vi "log analysis_gps.vi"() -> ()   [LabVIEW 2018] (continued)
0.1010,5.0842,0f000001,0*696fd9b1\n\t", "DUALANTENNAHEADINGA,USB3,0,48.5,FINESTEERING,2107,283554.100,02000000,d426,15824;INSUFFICIENT_OBS,NONE,-1.000000000,0.000000000,0.000000000,0.0,0.000000000,0.000000000,\"631T\",13,4,4,3,04,00,20,02*de32c05b\n\t", "INSPVAXA,USB3,0,51.0,FINESTEERING,2107,283554.600,02000000,471d,15824;INS_ALIGNMENT_COMPLETE,INS_RTKFIXED,37.37125848358,126.72235217781,7.9795,22.3000,0.0223,-0.2763,0.0124,-2.892819267,-0.280095971,268.699067349,0.4384,0.2951,0.5740,0.1126,0.0925,0.0783,0.0963,0.1010,5.0853,0f000001,0*82db867f\n\t", "DUALANTENNAHEADINGA,USB3,0,47.0,FINESTEERING,2107,283555.100,02000000,d426,15824;INSUFFICIENT_OBS,NONE,-1.000000000,0.000000000,0.000000000,0.0,0.000000000,0.000000000,\"631T\",14,4,4,3,04,00,20,03*a9c2070c\n\t", "INSPVAXA,USB3,0,47.0,FINESTEERING,2107,283555.600,02000000,471d,15824;INS_ALIGNMENT_COMPLETE,INS_RTKFIXED,37.37125853353,126.72234893237,7.9755,22.3000,0.0216,-0.2860,0.0144,-2.819506648,-0.407770491,269.082070244,0.4381,0.2951,0.5741,0.1126,0.0924,0.0783,0.0963,0.1010,5.0867,0f000001,0*4971d182\n\t", "INSPVAXA,USB3,0,45.0,FINESTEERING,2107,283556.100,02000000,471d,15824;INS_ALIGNMENT_COMPLETE,INS_RTKFIXED,37.37125856914,126.72234737250,7.9744,22.3000,0.0229,-0.2921,0.0135,-2.758204349,-0.398675406,269.289539292,0.4378,0.2952,0.5740,0.1126,0.0924,0.0783,0.0962,0.1010,5.0883,0f000001,0*04f4864c\n\t", "DUALANTENNAHEADINGA,USB3,0,45.0,FINESTEERING,2107,283556.600,02000000,d426,15824;INSUFFICIENT_OBS,NONE,-1.000000000,0.000000000,0.000000000,0.0,0.000000000,0.000000000,\"631T\",14,4,4,3,04,00,20,03*1b8bbdb9\n\t", "DUALANTENNAHEADINGA,USB3,0,45.0,FINESTEERING,2107,283557.100,02000000,d426,15824;INSUFFICIENT_OBS,NONE,-1.000000000,0.000000000,0.000000000,0.0,0.000000000,0.000000000,\"631T\",15,4,4,3,04,00,20,03*6d1923ae\n\t", "DUALANTENNAHEADINGA,USB3,0,46.5,FINESTEERING,2107,283557.600,02000000,d426,15824;INSUFFICIENT_OBS,NONE,-1.000000000,0.000000000,0.000000000,0.0,0.000000000,0.000000000,\"631T\",14,4,4,3,04,00,20,03*8fe42440\n\t", "DUALANTENNAHEADINGA,USB3,0,46.5,FINESTEERING,2107,283558.100,02000000,d426,15824;INSUFFICIENT_OBS,NONE,-1.000000000,0.000000000,0.000000000,0.0,0.000000000,0.000000000,\"631T\",11,4,4,3,04,00,20,02*089ab1fe\n\t", "INSPVAXA,USB3,0,47.5,FINESTEERING,2107,283558.600,02000000,471d,15824;INS_ALIGNMENT_COMPLETE,INS_RTKFIXED,37.37125886562,126.72233975708,7.9685,22.3000,0.0526,-0.2759,0.0211,-2.409557071,-0.340107874,269.967780628,0.4378,0.2950,0.5739,0.1125,0.0924,0.0783,0.0962,0.1009,5.0913,0f000001,0*5e667246\n\t", "DUALANTENNAHEADINGA,USB3,0,47.5,FINESTEERING,2107,283559.100,02008000,d426,15824;INSUFFICIENT_OBS,NONE,-1.000000000,0.000000000,0.000000000,0.0,0.000000000,0.000000000,\"631T\",9,4,4,3,04,00,20,03*5bfaaf18\n\t", "DUALANTENNAHEADINGA,USB3,0,51.0,FINESTEERING,2107,283559.600,02008000,d426,15824;INSUFFICIENT_OBS,NONE,-1.000000000,0.000000000,0.000000000,0.0,0.000000000,0.000000000,\"631T\",11,4,4,3,04,00,20,03*aa74f950\n\t", "DUALANTENNAHEADINGA,USB3,0,43.5,FINESTEERING,2107,283560.100,02008000,d426,15824;INSUFFICIENT_OBS,NONE,-1.000000000,0.000000000,0.000000000,0.0,0.000000000,0.000000000,\"631T\",12,4,4,3,04,00,20,02*918dc314\n\t", "INSPVAXA,USB3,0,43.5,FINESTEERING,2107,283560.600,02008000,471d,15824;INS_ALIGNMENT_COMPLETE,INS_RTKFIXED,37.37125922477,126.72233331539,7.9711,22.3000,0.0461,-0.3029,0.0142,-2.105523961,0.098116504,270.318274292,0.4374,0.2952,0.5740,0.1125,0.0925,0.0783,0.0962,0.1009,5.0942,0f000001,0*4e7a44d6\n\t", "DUALANTENNAHEADINGA,USB3,0,45.0,FINESTEERING,2107,283561.600,02008000,d426,15824;INSUFFICIENT_OBS,NONE,-1.000000000,0.000000000,0.000000000,0.0,0.000000000,0.000000000,\"631T\",11,4,4,3,04,00,20,03*333d7c31\n\t", "DUALANTENNAHEADINGA,USB3,0,45.0,FINESTEERING,2107,283562.100,02008000,d426,15824;INSUFFICIENT_OBS,NONE,-1.000000000,0.000000000,0.000000000,0.0,0.000000000,0.000000000,\"631T\",10,4,4,3,04,00,20,03*9e1feb94\n\t", "DUALANTENNAHEADINGA,USB3,0,49.5,FINESTEERING,2107,283562.600,02008000,d426,15824;INSUFFICIENT_OBS,NONE,-1.000000000,0.000000000,0.000000000,0.0,0.000000000,0.000000000,\"631T\",11,4,4,3,04,00,20,03*0e8972e5\n\t", "DUALANTENNAHEADINGA,USB3,0,49.5,FINESTEERING,2107,283563.100,02008000,d426,15824;INSUFFICIENT_OBS,NONE,-1.000000000,0.000000000,0.000000000,0.0,0.000000000,0.000000000,\"631T\",12,4,4,3,04,00,20,03*0cafea03\n\t", "DUALANTENNAHEADINGA,USB3,0,49.5,FINESTEERING,2107,283563.600,02000000,d426,15824;INSUFFICIENT_OBS,NONE,-1.000000000,0.000000000,0.000000000,0.0,0.000000000,0.000000000,\"631T\",11,4,4,3,04,00,20,03*75c2f29d\n\t", "DUALANTENNAHEADINGA,USB3,0,46.5,FINESTEERING,2107,283564.100,02000000,d426,15824;INSUFFICIENT_OBS,NONE,-1.000000000,0.000000000,0.000000000,0.0,0.000000000,0.000000000,\"631T\",12,4,4,3,04,00,20,03*b22ee873\n\t", "DUALANTENNAHEADINGA,USB3,0,46.5,FINESTEERING,2107,283564.600,02000000,d426,15824;INSUFFICIENT_OBS,NONE,-1.000000000,0.000000000,0.000000000,0.0,0.000000000,0.000000000,\"631T\",13,4,4,3,04,00,20,03*a96472bd\n\t", "DUALANTENNAHEADINGA,USB3,0,46.5,FINESTEERING,2107,283565.100,02000000,d426,15824;INSUFFICIENT_OBS,NONE,-1.000000000,0.000000000,0.000000000,0.0,0.000000000,0.000000000,\"631T\",13,4,4,3,04,00,20,03*08146cf2\n\t", "DUALANTENNAHEADINGA,USB3,0,48.0,FINESTEERING,2107,283565.600,02000000,d426,15824;INSUFFICIENT_OBS,NONE,-1.000000000,0.000000000,0.000000000,0.0,0.000000000,0.000000000,\"631T\",12,4,4,3,04,00,20,03*500b58cb\n\t", "DUALANTENNAHEADINGA,USB3,0,48.0,FINESTEERING,2107,283566.100,02000000,d426,15824;INSUFFICIENT_OBS,NONE,-1.000000000,0.000000000,0.000000000,0.0,0.000000000,0.000000000,\"631T\",13,4,4,3,04,00,20,02*8a2efff8\n\t", "INSPVAXA,USB3,0,47.0,FINESTEERING,2107,283567.150,02000000,471d,15824;INS_ALIGNMENT_COMPLETE,INS_RTKFIXED,37.37126023924,126.72231232835,7.9766,22.3000,0.0196,-0.2915,0.0203,-1.615683840,-0.184237550,266.738571120,0.4436,0.2960,0.5749,0.1133,0.0925,0.0784,0.0962,0.1011,5.1038,0f000001,0*2b446319\n\t", "DUALANTENNAHEADINGA,USB3,0,47.0,FINESTEERING,2107,283567.600,02000000,d426,15824;INSUFFICIENT_OBS,NONE,-1.000000000,0.000000000,0.000000000,0.0,0.000000000,0.000000000,\"631T\",12,4,4,3,04,00,20,02*8ed7ff70\n\t", "DUALANTENNAHEADINGA,USB3,0,47.0,FINESTEERING,2107,283568.100,02000000,d426,15824;INSUFFICIENT_OBS,NONE,-1.000000000,0.000000000,0.000000000,0.0,0.000000000,0.000000000,\"631T\",14,4,4,3,04,00,20,03*aaffec67\n\t", "INSPVAXA,USB3,0,50.5,FINESTEERING,2107,283568.650,02000000,471d,15824;INS_ALIGNMENT_COMPLETE,INS_RTKFIXED,37.37126026613,126.72230748127,7.9785,22.3000,0.0314,-0.2890,0.0136,-1.676303872,0.031387209,266.013991723,0.4441,0.2961,0.5750,0.1133,0.0925,0.0784,0.0962,0.1011,5.1051,0f000001,0*382c449f\n\t", "DUALANTENNAHEADINGA,USB3,0,40.0,FINESTEERING,2107,283569.100,02000000,d426,15824;INSUFFICIENT_OBS,NONE,-1.000000000,0.000000000,0.000000000,0.0,0.000000000,0.000000000,\"631T\",13,4,4,3,04,00,20,02*1cb1745e\n\t", "DUALANTENNAHEADINGA,USB3,0,40.0,FINESTEERING,2107,283569.600,02000000,d426,15824;INSUFFICIENT_OBS,NONE,-1.000000000,0.000000000,0.000000000,0.0,0.000000000,0.000000000,\"631T\",13,4,4,3,04,00,20,03*a71e5e5e\n\t", "INSPVAXA,USB3,0,51.0,FINESTEERING,2107,283570.150,02000000,471d,15824;INS_ALIGNMENT_COMPLETE,INS_RTKFIXED,37.37126027188,126.72230260848,7.9782,22.3000,0.0223,-0.2985,0.0040,-1.310118648,0.027956781,265.914374243,0.4449,0.2965,0.5753,0.1133,0.0927,0.0784,0.0962,0.1011,5.1080,0f000001,0*e4cc9c92\n\t", "INSPVAXA,USB3,0,51.0,FINESTEERING,2107,283570.650,02000000,471d,15824;INS_ALIGNMENT_COMPLETE,INS_RTKFIXED,37.37126026750,126.72230111428,7.9776,22.3000,0.0310,-0.1470,0.0080,-1.255276150,-0.174138807,265.875286689,0.4449,0.2965,0.5753,0.1133,0.0927,0.0784,0.0962,0.1011,5.1080,0f000001,0*fb01e8e4\n\t", "INSPVAXA,USB3,0,50.0,FINESTEERING,2107,283571.150,02000000,471d,15824;INS_ALIGNMENT_COMPLETE,INS_RTKFIXED,37.37126027111,126.72229951558,7.9776,22.3000,-0.0095,-0.3504,-0.0012,-1.130419534,-0.185484043,265.929537810,0.4449,0.2965,0.5753,0.1133,0.0927,0.0784,0.0962,0.1011,5.1080,0f000001,0*20782363\n\t", "DUALANTENNAHEADINGA,USB3,0,50.0,FINESTEERING,2107,283572.100,02000000,d426,15824;INSUFFICIENT_OBS,NONE,0.000000000,0.000000000,0.000000000,0.0,0.000000000,0.000000000,\"\",0,0,0,0,00,00,00,00*5d8535fc\n\t", "DUALANTENNAHEADINGA,USB3,0,52.5,FINESTEERING,2107,283572.600,02000000,d426,15824;INSUFFICIENT_OBS,NONE,0.000000000,0.000000000,0.000000000,0.0,0.000000000,0.000000000,\"\",0,0,0,0,00,00,00,00*859f07a2\n\t", "DUALANTENNAHEADINGA,USB3,0,50.0,FINESTEERING,2107,283573.100,02000000,d426,15824;INSUFFICIENT_OBS,NONE,0.000000000,0.000000000,0.000000000,0.0,0.000000000,0.000000000,\"\",0,0,0,0,00,00,00,00*a797c2ea\n\t", "INSPVAXA,USB3,0,52.0,FINESTEERING,2107,283574.650,02000000,471d,15824;INS_ALIGNMENT_COMPLETE,INS_RTKFIXED,37.37126025479,126.72228822591,7.9861,22.3000,0.0090,-0.3026,-0.0003,-0.524199220,-0.126443269,266.389234836,0.4991,0.3317,0.6500,0.1205,0.0986,0.0804,0.0985,0.1030,5.1132,0f000001,0*c3c99d89\n\t", "INSPVAXA,USB3,0,50.0,FINESTEERING,2107,283575.150,02000000,471d,15824;INS_ALIGNMENT_COMPLETE,INS_RTKFIXED,37.37126023129,126.72228662486,7.9852,22.3000,0.0085,-0.2932,0.0017,-0.596688743,-0.097225443,266.485321234,0.4751,0.3142,0.6322,0.1185,0.0977,0.0789,0.0982,0.1027,5.1147,0f000001,0*e174b094\n\t", "INSPVAXA,USB3,0,50.0,FINESTEERING,2107,283575.650,02000000,471d,15824;INS_ALIGNMENT_COMPLETE,INS_RTKFIXED,37.37126022571,126.72228518067,7.9842,22.3000,-0.0010,-0.2887,0.0210,-0.683424263,-0.147084143,266.527685008,0.4751,0.3142,0.6322,0.1185,0.0977,0.0789,0.0982,0.1027,5.1147,0f000001,0*c2e268d1\n\t", "INSPVAXA,USB3,0,50.0,FINESTEERING,2107,283576.150,02000000,471d,15824;INS_ALIGNMENT_COMPLETE,INS_RTKFIXED,37.37126021633,126.72228346240,7.9840,22.3000,0.0021,-0.2751,0.0114,-0.667866815,-0.315367181,266.708831075,0.4606,0.3053,0.6179,0.1181,0.0979,0.0781,0.0979,0.1024,5.1163,0f000001,0*0ba78e3d\n\t", "INSPVAXA,USB3,0,50.0,FINESTEERING,2107,283576.650,02000000,471d,15824;INS_ALIGNMENT_COMPLETE,INS_RTKFIXED,37.37126022512,126.72228190722,7.9848,22.3000,-0.0006,-0.2994,0.0229,-0.670999350,-0.155338039,266.786409078,0.4606,0.3053,0.6179,0.1181,0.0979,0.0781,0.0979,0.1024,5.1163,0f000001,0*9811c325\n\t", "INSPVAXA,USB3,0,48.5,FINESTEERING,2107,283577.650,02000000,471d,15824;INS_ALIGNMENT_COMPLETE,INS_RTKFIXED,37.37126026454,126.72227868899,7.9856,22.3000,0.0080,-0.2785,0.0173,-0.609374053,-0.154098562,267.060666338,0.4521,0.3012,0.6064,0.1181,0.0980,0.0776,0.0975,0.1023,5.1178,0f000001,0*aa9c2bc5\n\t", "INSPVAXA,USB3,0,51.5,FINESTEERING,2107,283579.150,02000000,471d,15824;INS_ALIGNMENT_COMPLETE,INS_RTKFIXED,37.37126037410,126.72227378516,7.9904,22.3000,0.0163,-0.2830,0.0173,-0.746603441,-0.380752059,267.626447850,0.4463,0.2992,0.5904,0.1180,0.0971,0.0775,0.0966,0.1018,5.1209,0f000001,0*da9a51df\n\t", "INSPVAXA,USB3,0,51.5,FINESTEERING,2107,283579.650,02000000,471d,15824;INS_ALIGNMENT_COMPLETE,INS_RTKFIXED,37.37126042399,126.72227213267,7.9925,22.3000,0.0129,-0.2940,0.0192,-0.723337751,-0.333271037,267.787526970,0.4463,0.2992,0.5904,0.1180,0.0971,0.0775,0.0966,0.1018,5.1209,0f000001,0*2d4308ff\n\t", "INSPVAXA,USB3,0,52.5,FINESTEERING,2107,283580.150,02000000,471d,15824;INS_ALIGNMENT_COMPLETE,INS_RTKFIXED,37.37126049043,126.72227055501,7.9950,22.3000,0.0243,-0.3033,0.0180,-0.573377117,-0.330323438,267.951447700,0.4448,0.2989,0.5852,0.1175,0.0961,0.0776,0.0961,0.1014,5.1224,0f000001,0*65285ec1\n\t", "DUALANTENNAHEADINGA,USB3,0,48.0,FINESTEERING,2107,283581.100,02000000,d426,15824;INSUFFICIENT_OBS,NONE,0.000000000,0.000000000,0.000000000,0.0,0.000000000,0.000000000,\"\",0,0,0,0,00,00,00,00*0d472a41\n\t", "INSPVAXA,USB3,0,48.0,FINESTEERING,2107,283581.650,02000000,471d,15824;INS_ALIGNMENT_COMPLETE,INS_RTKFIXED,37.37126070396,126.72226577509,8.0028,22.3000,0.0230,-0.2933,0.0344,-0.578760971,-0.170041590,268.380757067,0.4441,0.2986,0.5812,0.1168,0.0951,0.0777,0.0958,0.1011,5.1238,0f000001,0*94c5c4b2\n\t", "INSPVAXA,USB3,0,50.0,FINESTEERING,2107,283582.650,02000000,471d,15824;INS_ALIGNMENT_COMPLETE,INS_RTKFIXED,37.37126086300,126.72226255094,8.0114,22.3000,0.0186,-0.2902,0.0297,-0.554451124,-0.113657827,268.567093928,0.4437,0.2982,0.5783,0.1160,0.0941,0.0779,0.0956,0.1009,5.1252,0f000001,0*de1d38ac\n\t", "INSPVAXA,USB3,0,52.0,FINESTEERING,2107,283583.150,02000000,471d,15824;INS_ALIGNMENT_COMPLETE,INS_RTKFIXED,37.37126094107,126.72226089314,8.0147,22.3000,0.0176,-0.2816,0.0224,-0.681553326,-0.108375043,268.657687253,0.4431,0.2976,0.5763,0.1151,0.0933,0.0781,0.0955,0.1007,5.1266,0f000001,0*8a630b8d\n\t", "INSPVAXA,USB3,0,52.0,FINESTEERING,2107,283583.650,02000000,471d,15824;INS_ALIGNMENT_COMPLETE,INS_RTKFIXED,37.37126102705,126.72225926038,8.0174,22.3000,0.0194,-0.3033,0.0147,-0.616207417,-0.286762817,268.672715403,0.4431,0.2976,0.5763,0.1151,0.0933,0.0781,0.0955,0.1007,5.1266,0f000001,0*61848793\n\t", "INSPVAXA,USB3,0,52.0,FINESTEERING,2107,283584.150,02000000,471d,15824;INS_ALIGNMENT_COMPLETE,INS_RTKFIXED,37.37126112105,126.72225762489,8.0208,22.3000,0.0251,-0.2868,0.0143,-0.484996115,-0.348090113,268.682050647,0.4426,0.2969,0.5750,0.1144,0.0927,0.0782,0.0955,0.1006,5.1279,0f000001,0*d30f3e54\n\t", "INSPVAXA,USB3,0,52.0,FINESTEERING,2107,283584.650,02000000,471d,15824;INS_ALIGNMENT_COMPLETE,INS_RTKFIXED,37.37126121621,126.72225620166,8.0227,22.3000,0.0321,-0.0816,0.0199,-0.459149355,-0.498683965,268.628376377,0.4426,0.2969,0.5750,0.1144,0.0927,0.0782,0.0955,0.1006,5.1279,0f000001,0*e5ed7c63\n\t", "INSPVAXA,USB3,0,49.0,FINESTEERING,2107,283585.150,02000000,471d,15824;INS_ALIGNMENT_COMPLETE,INS_RTKFIXED,37.37126129698,126.72225459849,8.0251,22.3000,0.0349,-0.3426,0.0329,-0.569349800,-0.560640511,268.532383253,0.4425,0.2966,0.5744,0.1144,0.0924,0.0784,0.0956,0.1006,5.1294,0f000001,0*4640cbf6\n\t", "INSPVAXA,USB3,0,49.0,FINESTEERING,2107,283585.650,02000000,471d,15824;INS_ALIGNMENT_COMPLETE,INS_RTKFIXED,37.37126137394,126.72225308543,8.0277,22.3000,0.0305,-0.3477,0.0168,-0.707352535,-0.516144165,268.333596331,0.4425,0.2966,0.5744,0.1144,0.0924,0.0784,0.0956,0.1006,5.1294,0f000001,0*ea5ffab2\n\t", "INSPVAXA,USB3,0,50.5,FINESTEERING,2107,283586.150,02000000,471d,15824;INS_ALIGNMENT_COMPLETE,INS_RTKFIXED,37.37126146482,126.72225147889,8.0290,22.3000,0.0318,-0.3117,0.0162,-0.540726540,-0.516678625,268.023762114,0.4406,0.2960,0.5741,0.1134,0.0922,0.0785,0.0957,0.1006,5.1306,0f000001,0*2ae37417\n\t", "INSPVAXA,USB3,0,50.5,FINESTEERING,2107,283586.650,02000000,471d,15824;INS_ALIGNMENT_COMPLETE,INS_RTKFIXED,37.37126154442,126.72224983237,8.0302,22.3000,0.0153,-0.2976,0.0132,-0.405221817,-0.801510438,267.749524136,0.4406,0.2960,0.5741,0.1134,0.0922,0.0785,0.0957,0.1006,5.1306,0f000001,0*889b905c\n\t", "INSPVAXA,USB3,0,48.5,FINESTEERING,2107,283587.150,02000000,471d,15824;INS_ALIGNMENT_COMPLETE,INS_RTKFIXED,37.37126161078,126.72224818389,8.0314,22.3000,0.0135,-0.2861,0.0058,-0.357423684,-1.016170306,267.360005702,0.4401,0.2956,0.5740,0.1128,0.0921,0.0786,0.0958,0.1006,5.1321,0f000001,0*b354eb89\n\t", "DUALANTENNAHEADINGA,USB3,0,48.5,FINESTEERING,2107,283587.600,02000000,d426,15824;INSUFFICIENT_OBS,NONE,0.000000000,0.000000000,0.000000000,0.0,0.000000000,0.000000000,\"\",0,0,0,0,00,00,00,00*3e024a6f\n\t", "INSPVAXA,USB3,0,49.5,FINESTEERING,2107,283588.650,02000000,471d,15824;INS_ALIGNMENT_COMPLETE,INS_RTKFIXED,37.37126174157,126.72224330005,8.0321,22.3000,0.0403,-0.2838,0.0098,-0.134470490,-1.230467800,265.991496419,0.4395,0.2955,0.5741,0.1126,0.0921,0.0786,0.0959,0.1007,5.1336,0f000001,0*86c47da8\n\t", "INSPVAXA,USB3,0,51.5,FINESTEERING,2107,283589.150,02000000,471d,15824;INS_ALIGNMENT_COMPLETE,INS_RTKFIXED,37.37126177483,126.72224169465,8.0328,22.3000,0.0428,-0.2922,0.0200,-0.044724950,-0.991745549,265.567471181,0.4384,0.2954,0.5742,0.1124,0.0922,0.0786,0.0960,0.1008,5.1352,0f000001,0*fd2974d4\n\t", "INSPVAXA,USB3,0,51.5,FINESTEERING,2107,283589.650,02000000,471d,15824;INS_ALIGNMENT_COMPLETE,INS_RTKFIXED,37.37126179570,126.72224014857,8.0325,22.3000,0.0430,-0.3072,0.0249,-0.007617366,-0.680507333,265.196792969,0.4384,0.2954,0.5742,0.1124,0.0922,0.0786,0.0960,0.1008,5.1352,0f000001,0*75474069\n\t", "INSPVAXA,USB3,0,52.0,FINESTEERING,2107,283590.150,02000000,471d,15824;INS_ALIGNMENT_COMPLETE,INS_RTKFIXED,37.37126181306,126.72223852203,8.0321,22.3000,0.0371,-0.3064,0.0221,-0.054866167,-0.319461022,264.939008114,0.4379,0.2954,0.5744,0.1124,0.0922,0.0786,0.0960,0.1008,5.1368,0f000001,0*489db8a8\n\t", "INSPVAXA,USB3,0,52.0,FINESTEERING,2107,283590.650,02000000,471d,15824;INS_ALIGNMENT_COMPLETE,INS_RTKFIXED,37.37126182845,126.72223689511,8.0304,22.3000,0.0329,-0.2983,0.0263,-0.099615260,-0.144209123,264.670119268,0.4379,0.2954,0.5744,0.1124,0.0922,0.0786,0.0960,0.1008,5.1368,0f000001,0*3ff0cb58\n\t", "INSPVAXA,USB3,0,46.5,FINESTEERING,2107,283591.650,02000000,471d,15824;INS_ALIGNMENT_COMPLETE,INS_RTKFIXED,37.37126184009,126.72223359143,8.0280,22.3000,0.0242,-0.3040,0.0144,-0.139661559,-0.269205347,264.433455917,0.4387,0.2955,0.5748,0.1127,0.0923,0.0786,0.0961,0.1009,5.1382,0f000001,0*bb357185\n\t", "INSPVAXA,USB3,0,50.0,FINESTEERING,2107,283592.150,02000000,471d,15824;INS_ALIGNMENT_COMPLETE,INS_RTKFIXED,37.37126183340,126.72223190361,8.0268,22.3000,0.0217,-0.3070,0.0246,-0.250767704,-0.520528814,264.430385141,0.4392,0.2956,0.5751,0.1125,0.0924,0.0786,0.0961,0.1010,5.1393,0f000001,0*012bab97\n\t", "INSPVAXA,USB3,0,50.0,FINESTEERING,2107,283592.650,02000000,471d,15824;INS_ALIGNMENT_COMPLETE,INS_RTKFIXED,37.37126182669,126.72223026122,8.0254,22.3000,0.0249,-0.2956,0.0206,-0.309442980,-0.761179345,264.440443486,0.4392,0.2956,0.5751,0.1125,0.0924,0.0786,0.0961,0.1010,5.1393,0f000001,0*78c848e1\n\t", "INSPVAXA,USB3,0,44.5,FINESTEERING,2107,283593.650,02000000,471d,15824;INS_ALIGNMENT_COMPLETE,INS_RTKFIXED,37.37126179813,126.72222695533,8.0221,22.3000,0.0365,-0.2965,0.0185,-0.369051929,-1.148324870,264.580362201,0.4393,0.2956,0.5754,0.1125,0.0925,0.0786,0.0962,0.1010,5.1403,0f000001,0*8be4a412\n\t", "INSPVAXA,USB3,0,43.0,FINESTEERING,2107,283594.150,02000000,471d,15824;INS_ALIGNMENT_COMPLETE,INS_RTKFIXED,37.37126178881,126.72222531638,8.0209,22.3000,0.0318,-0.2892,0.0117,-0.315197782,-1.127826299,264.669850736,0.4395,0.2956,0.5757,0.1126,0.0925,0.0786,0.0962,0.1010,5.1415,0f000001,0*2d917e72\n\t", "INSPVAXA,USB3,0,43.0,FINESTEERING,2107,283594.650,02000000,471d,15824;INS_ALIGNMENT_COMPLETE,INS_RTKFIXED,37.37126177423,126.72222371508,8.0192,22.3000,0.0303,-0.3062,0.0087,-0.244943668,-0.998392292,264.739545635,0.4395,0.2956,0.5757,0.1126,0.0925,0.0786,0.0962,0.1010,5.1415,0f000001,0*36684632\n\t", "INSPVAXA,USB3,0,48.0,FINESTEERING,2107,283595.150,02000000,471d,15824;INS_ALIGNMENT_COMPLETE,INS_RTKFIXED,37.37126177448,126.72222209651,8.0178,22.3000,0.0339,-0.2977,0.0111,-0.119926645,-0.839441888,264.806746859,0.4396,0.2957,0.5758,0.1127,0.0925,0.0786,0.0962,0.1011,5.1428,0f000001,0*08adb1ac\n\t", "INSPVAXA,USB3,0,48.0,FINESTEERING,2107,283595.650,02000000,471d,15824;INS_ALIGNMENT_COMPLETE,INS_RTKFIXED,37.37126175579,126.72222044305,8.0158,22.3000,0.0315,-0.2901,0.0146,-0.140682450,-0.757275423,264.939327324,0.4396,0.2957,0.5758,0.1127,0.0925,0.0786,0.0962,0.1011,5.1428,0f000001,0*78aa4323\n\t", "INSPVAXA,USB3,0,45.5,FINESTEERING,2107,283596.150,02000000,471d,15824;INS_ALIGNMENT_COMPLETE,INS_RTKFIXED,37.37126174706,126.72221882268,8.0135,22.3000,0.0328,-0.3087,0.0055,-0.159363223,-0.689273148,265.030991748,0.4393,0.2956,0.5759,0.1126,0.0925,0.0785,0.0962,0.1010,5.1440,0f000001,0*bc7a17e4\n\t", "INSPVAXA,USB3,0,47.0,FINESTEERING,2107,283597.650,02000000,471d,15824;INS_ALIGNMENT_COMPLETE,INS_RTKFIXED,37.37126174585,126.72221399388,8.0051,22.3000,0.0336,-0.3137,-0.0021,0.019465738,-0.716944354,265.373596079,0.4393,0.2957,0.5759,0.1127,0.0925,0.0785,0.0962,0.1010,5.1453,0f000001,0*fd9fbe4c\n\t", "INSPVAXA,USB3,0,50.5,FINESTEERING,2107,283598.150,02000000,471d,15824;INS_ALIGNMENT_COMPLETE,INS_RTKFIXED,37.37126175152,126.72221241027,8.0034,22.3000,0.0326,-0.3115,-0.0006,-0.014551220,-0.589641139,265.465982891,0.4393,0.2958,0.5760,0.1127,0.0925,0.0785,0.0962,0.1010,5.1467,0f000001,0*f52d235f\n\t", "INSPVAXA,USB3,0,50.5,FINESTEERING,2107,283598.650,02000000,471d,15824;INS_ALIGNMENT_COMPLETE,INS_RTKFIXED,37.37126174603,126.72221081507,8.0012,22.3000,0.0404,-0.2514,0.0050,0.007312732,-0.531763508,265.590138557,0.4393,0.2958,0.5760,0.1127,0.0925,0.0785,0.0962,0.1010,5.1467,0f000001,0*8824c4d8\n\t", "INSPVAXA,USB3,0,47.5,FINESTEERING,2107,283599.150,02000000,471d,15824;INS_ALIGNMENT_COMPLETE,INS_RTKFIXED,37.37126176062,126.72220950725,7.9992,22.3000,0.0252,-0.3434,0.0010,0.008395245,-0.454774563,265.666808103,0.4392,0.2959,0.5760,0.1129,0.0925,0.0784,0.0962,0.1010,5.1480,0f000001,0*d239d7e1\n\t", "INSPVAXA,USB3,0,49.0,FINESTEERING,2107,283600.150,02000000,471d,15824;INS_ALIGNMENT_COMPLETE,INS_RTKFIXED,37.37126175398,126.72220624813,7.9941,22.3000,0.0263,-0.2975,0.0106,0.196462892,-0.509026578,265.990503300,0.4393,0.2959,0.5760,0.1126,0.0926,0.0784,0.0962,0.1010,5.1489,0f000001,0*3b9f52b7\n\t", "INSPVAXA,USB3,0,49.0,FINESTEERING,2107,283601.150,02000000,471d,15824;INS_ALIGNMENT_COMPLETE,INS_RTKFIXED,37.37126176703,126.72220301301,7.9883,22.3000,0.0322,-0.3028,0.0049,0.082285729,-0.304157914,266.276129441,0.4386,0.2961,0.5760,0.1125,0.0925,0.0784,0.0962,0.1009,5.1498,0f000001,0*cfc5bf1f\n\t", "INSPVAXA,USB3,0,49.0,FINESTEERING,2107,283601.650,02000000,471d,15824;INS_ALIGNMENT_COMPLETE,INS_RTKFIXED,37.37126177893,126.72220143158,7.9847,22.3000,0.0347,-0.3053,0.0090,0.167695581,-0.286452712,266.390208904,0.4386,0.2961,0.5760,0.1125,0.0925,0.0784,0.0962,0.1009,5.1498,0f000001,0*1c01ffd1\n\t", "INSPVAXA,USB3,0,50.0,FINESTEERING,2107,283602.150,02000000,471d,15824;INS_ALIGNMENT_COMPLETE,INS_RTKFIXED,37.37126180222,126.72219979604,7.9806,22.3000,0.0339,-0.2918,-0.0010,0.296365252,-0.279449744,266.507882837,0.4383,0.2960,0.5760,0.1125,0.0926,0.0784,0.0962,0.1009,5.1509,0f000001,0*8cd233aa\n\t", "INSPVAXA,USB3,0,50.5,FINESTEERING,2107,283604.650,02000000,471d,15824;INS_ALIGNMENT_COMPLETE,INS_RTKFIXED,37.37126199805,126.72219243143,7.9649,22.3000,0.0555,0.0695,0.0079,0.560896506,-1.435960650,267.028457385,0.4379,0.2961,0.5759,0.1131,0.0925,0.0784,0.0963,0.1009,5.1528,0f000001,0*81aa449e\n\t", "INSPVAXA,USB3,0,45.0,FINESTEERING,2107,283607.150,02000000,471d,15824;INS_ALIGNMENT_COMPLETE,INS_RTKFIXED,37.37126226214,126.72219256337,7.9563,22.3000,0.0507,-0.0122,0.0067,0.527133772,-1.343948140,267.105174531,0.4402,0.2962,0.5756,0.1140,0.0925,0.0784,0.0963,0.1009,5.1518,0f000001,0*37532215\n\t", "INSPVAXA,USB3,0,45.0,FINESTEERING,2107,283607.650,02000000,471d,15824;INS_ALIGNMENT_COMPLETE,INS_RTKFIXED,37.37126225847,126.72219257288,7.9545,22.3000,0.0487,-0.0117,0.0063,0.526769970,-1.341614130,267.120484585,0.4402,0.2962,0.5756,0.1140,0.0925,0.0784,0.0963,0.1009,5.1518,0f000001,0*097e3cbc\n\t", "INSPVAXA,USB3,0,49.5,FINESTEERING,2107,283619.700,02000000,471d,15824;INS_ALIGNMENT_COMPLETE,INS_RTKFIXED,37.37126206039,126.72216378783,7.9456,22.3000,0.0422,-0.2948,0.0158,1.718323220,-0.193748450,266.266037782,0.4350,0.2957,0.5763,0.1125,0.0925,0.0784,0.0965,0.1009,5.1330,0f000001,0*8635b490\n\t", "INSPVAXA,USB3,0,47.5,FINESTEERING,2107,283622.200,02000000,471d,15824;INS_ALIGNMENT_COMPLETE,INS_RTKFIXED,37.37126217486,126.72215605148,7.9488,22.3000,0.0265,-0.2568,0.0016,0.953197769,-0.264991418,265.735651965,0.4362,0.2956,0.5763,0.1134,0.0927,0.0784,0.0965,0.1010,5.1347,0f000001,0*d1c7aea0\n\t", "INSPVAXA,USB3,0,49.5,FINESTEERING,2107,283623.200,02000000,471d,15824;INS_ALIGNMENT_COMPLETE,INS_RTKFIXED,37.37126215352,126.72215258792,7.9480,22.3000,0.0351,-0.2613,0.0231,0.659350525,-0.553290360,265.516937653,0.4377,0.2954,0.5765,0.1123,0.0931,0.0784,0.0965,0.1010,5.1353,0f000001,0*f37e3ed0\n\t", "INSPVAXA,USB3,0,49.5,FINESTEERING,2107,283625.200,02000000,471d,15824;INS_ALIGNMENT_COMPLETE,INS_RTKFIXED,37.37126210638,126.72214606046,7.9447,22.3000,0.0217,-0.2754,0.0073,0.236515804,-0.792213520,265.180407825,0.4366,0.2950,0.5766,0.1123,0.0931,0.0784,0.0964,0.1010,5.1329,0f000001,0*acc95a4e\n\t", "INSPVAXA,USB3,0,49.5,FINESTEERING,2107,283625.700,02000000,471d,15824;INS_ALIGNMENT_COMPLETE,INS_RTKFIXED,37.37126208247,126.72214443464,7.9445,22.3000,0.0140,-0.2813,0.0048,0.046048670,-0.588797871,265.114785763,0.4366,0.2950,0.5766,0.1123,0.0931,0.0784,0.0964,0.1010,5.1329,0f000001,0*ce0a2a96\n\t", "INSPVAXA,USB3,0,48.0,FINESTEERING,2107,283626.200,02000000,471d,15824;INS_ALIGNMENT_COMPLETE,INS_RTKFIXED,37.37126206372,126.72214280060,7.9445,22.3000,0.0212,-0.2855,0.0048,-0.004156486,-0.311026110,265.065225665,0.4366,0.2949,0.5766,0.1123,0.0931,0.0784,0.0963,0.1010,5.1300,0f000001,0*7442e942\n\t", "INSPVAXA,USB3,0,48.5,FINESTEERING,2107,283627.200,02000000,471d,15824;INS_ALIGNMENT_COMPLETE,INS_RTKFIXED,37.37126201142,126.72213963218,7.9431,22.3000,0.0278,-0.2914,0.0131,-0.197757356,0.430555181,264.900646420,0.4366,0.2949,0.5768,0.1127,0.0931,0.0784,0.0962,0.1009,5.1266,0f000001,0*c875f714\n\t", "INSPVAXA,USB3,0,48.0,FINESTEERING,2107,283628.700,02000000,471d,15824;INS_ALIGNMENT_COMPLETE,INS_RTKFIXED,37.37126191178,126.72213473323,7.9380,22.3000,0.0177,-0.2797,-0.0032,-0.623534384,0.011887408,264.986854356,0.4375,0.2949,0.5768,0.1127,0.0930,0.0784,0.0962,0.1009,5.1221,0f000001,0*2b23c567\n\t", "INSPVAXA,USB3,0,44.0,FINESTEERING,2107,283629.200,02000000,471d,15824;INS_ALIGNMENT_COMPLETE,INS_RTKFIXED,37.37126187751,126.72213308389,7.9364,22.3000,0.0207,-0.2899,-0.0036,-0.719101472,-0.426401600,265.021502859,0.4380,0.2949,0.5768,0.1123,0.0930,0.0784,0.0961,0.1009,5.1171,0f000001,0*92ebbc5f\n\t", "INSPVAXA,USB3,0,44.0,FINESTEERING,2107,283629.700,02000000,471d,15824;INS_ALIGNMENT_COMPLETE,INS_RTKFIXED,37.37126184367,126.72213142920,7.9356,22.3000,0.0231,-0.2981,-0.0100,-0.725013495,-0.732992105,265.121442983,0.4380,0.2949,0.5768,0.1123,0.0930,0.0784,0.0961,0.1009,5.1171,0f000001,0*6a5775b3\n\t", "INSPVAXA,USB3,0,47.0,FINESTEERING,2107,283630.200,02000000,471d,15824;INS_ALIGNMENT_COMPLETE,INS_RTKFIXED,37.37126181957,126.72212981940,7.9352,22.3000,0.0233,-0.2888,-0.0019,-0.675781239,-0.810566304,265.160131093,0.4376,0.2949,0.5768,0.1123,0.0928,0.0784,0.0961,0.1009,5.1128,0f000001,0*27ca04ea\n\t", "INSPVAXA,USB3,0,47.0,FINESTEERING,2107,283630.700,02000000,471d,15824;INS_ALIGNMENT_COMPLETE,INS_RTKFIXED,37.37126178591,126.72212819473,7.9347,22.3000,0.0150,-0.2861,-0.0012,-0.714770911,-0.869266848,265.221494891,0.4376,0.2949,0.5768,0.1123,0.0928,0.0784,0.0961,0.1009,5.1128,0f000001,0*aed2de40\n\t", "INSPVAXA,USB3,0,42.0,FINESTEERING,2107,283631.200,02000000,471d,15824;INS_ALIGNMENT_COMPLETE,INS_RTKFIXED,37.37126175832,126.72212651988,7.9323,22.3000,0.0193,-0.2829,-0.0000,-0.656726245,-0.814467356,265.316189024,0.4372,0.2950,0.5769,0.1123,0.0926,0.0784,0.0961,0.1009,5.1101,0f000001,0*d1b6c699\n\t", "INSPVAXA,USB3,0,42.0,FINESTEERING,2107,283631.700,02000000,471d,15824;INS_ALIGNMENT_COMPLETE,INS_RTKFIXED,37.37126176860,126.72212533305,7.9296,22.3000,0.0361,-0.3378,-0.0103,-0.428138119,-0.668837581,265.144757660,0.4372,0.2950,0.5769,0.1123,0.0926,0.0784,0.0961,0.1009,5.1101,0f000001,0*53a99c66\n\t", "INSPVAXA,USB3,0,48.5,FINESTEERING,2107,283632.700,02000000,471d,15824;INS_ALIGNMENT_COMPLETE,INS_RTKFIXED,37.37126172516,126.72212196595,7.9217,22.3000,0.0261,-0.3154,-0.0017,-0.080275609,-1.010698207,265.307907457,0.4366,0.2951,0.5768,0.1127,0.0925,0.0784,0.0961,0.1008,5.1091,0f000001,0*c955826f\n\t", "INSPVAXA,USB3,0,44.5,FINESTEERING,2107,283633.200,02000000,471d,15824;INS_ALIGNMENT_COMPLETE,INS_RTKFIXED,37.37126169079,126.72212014716,7.9199,22.3000,0.0199,-0.3002,0.0131,-0.062381377,-1.283391784,265.467989015,0.4356,0.2952,0.5768,0.1125,0.0925,0.0784,0.0961,0.1008,5.1096,0f000001,0*29ba6107\n\t", "INSPVAXA,USB3,0,44.5,FINESTEERING,2107,283633.700,02000000,471d,15824;INS_ALIGNMENT_COMPLETE,INS_RTKFIXED,37.37126167129,126.72211861960,7.9201,22.3000,0.0266,-0.3162,-0.0026,-0.118708398,-1.041509272,265.462110158,0.4356,0.2952,0.5768,0.1125,0.0925,0.0784,0.0961,0.1008,5.1096,0f000001,0*f2130a3a\n\t", "INSPVAXA,USB3,0,50.5,FINESTEERING,2107,283634.200,02000000,471d,15824;INS_ALIGNMENT_COMPLETE,INS_RTKFIXED,37.37126166951,126.72211687193,7.9193,22.3000,0.0345,-0.2873,0.0162,0.231523125,-0.963780299,265.599746817,0.4352,0.2955,0.5769,0.1123,0.0929,0.0784,0.0961,0.1009,5.1105,0f000001,0*34468b3e\n\t", "INSPVAXA,USB3,0,50.5,FINESTEERING,2107,283634.700,02000000,471d,15824;INS_ALIGNMENT_COMPLETE,INS_RTKFIXED,37.37126165383,126.72211529605,7.9180,22.3000,0.0293,-0.3222,-0.0026,0.312038300,-0.626564523,265.688696868,0.4352,0.2955,0.5769,0.1123,0.0929,0.0784,0.0961,0.1009,5.1105,0f000001,0*7451a5d1\n\t", "INSPVAXA,USB3,0,48.5,FINESTEERING,2107,283635.200,02000000,471d,15824;INS_ALIGNMENT_COMPLETE,INS_RTKFIXED,37.37126163429,126.72211368866,7.9175,22.3000,0.0223,-0.3021,-0.0082,0.186097207,-0.250317479,265.804263291,0.4352,0.2960,0.5769,0.1124,0.0928,0.0784,0.0961,0.1009,5.1109,0f000001,0*57ac3a22\n\t", "INSPVAXA,USB3,0,48.5,FINESTEERING,2107,283635.700,02000000,471d,15824;INS_ALIGNMENT_COMPLETE,INS_RTKFIXED,37.37126159822,126.72211206599,7.9179,22.3000,0.0256,-0.3005,0.0044,-0.110995339,-0.087789516,265.935244450,0.4352,0.2960,0.5769,0.1124,0.0928,0.0784,0.0961,0.1009,5.1109,0f000001,0*fb1bd604\n\t", "INSPVAXA,USB3,0,43.0,FINESTEERING,2107,283636.700,02000000,471d,15824;INS_ALIGNMENT_COMPLETE,INS_RTKFIXED,37.37126158491,126.72210906167,7.9172,22.3000,0.0261,-0.3515,0.0074,-0.153804874,-0.423258614,266.149623913,0.4359,0.2963,0.5769,0.1124,0.0927,0.0784,0.0961,0.1009,5.1114,0f000001,0*20701ae8\n\t", "INSPVAXA,USB3,0,48.5,FINESTEERING,2107,283637.200,02000000,471d,15824;INS_ALIGNMENT_COMPLETE,INS_RTKFIXED,37.37126157389,126.72210741579,7.9182,22.3000,0.0244,-0.2694,0.0184,-0.300056136,-0.600225307,266.307903185,0.4364,0.2964,0.5768,0.1122,0.0926,0.0784,0.0961,0.1009,5.1119,0f000001,0*6c5dc01c\n\t", "INSPVAXA,USB3,0,48.5,FINESTEERING,2107,283637.700,02000000,471d,15824;INS_ALIGNMENT_COMPLETE,INS_RTKFIXED,37.37126156174,126.72210572455,7.9205,22.3000,0.0137,-0.2979,0.0107,-0.519565417,-0.746251495,266.511093088,0.4364,0.2964,0.5768,0.1122,0.0926,0.0784,0.0961,0.1009,5.1119,0f000001,0*d93f2085\n\t", "INSPVAXA,USB3,0,51.0,FINESTEERING,2107,283638.200,02000000,471d,15824;INS_ALIGNMENT_COMPLETE,INS_RTKFIXED,37.37126155440,126.72210403454,7.9211,22.3000,0.0270,-0.3337,0.0126,-0.860556856,-0.781571793,266.718697356,0.4367,0.2965,0.5770,0.1123,0.0925,0.0784,0.0961,0.1009,5.1124,0f000001,0*3b4b6ae8\n\t", "INSPVAXA,USB3,0,51.0,FINESTEERING,2107,283638.700,02000000,471d,15824;INS_ALIGNMENT_COMPLETE,INS_RTKFIXED,37.37126156669,126.72210242363,7.9200,22.3000,0.0334,-0.3133,0.0178,-0.896958447,-0.619411990,266.906112882,0.4367,0.2965,0.5770,0.1123,0.0925,0.0784,0.0961,0.1009,5.1124,0f000001,0*cef03a1f\n\t", "INSPVAXA,USB3,0,50.0,FINESTEERING,2107,283639.200,02000000,471d,15824;INS_ALIGNMENT_COMPLETE,INS_RTKFIXED,37.37126157899,126.72210075579,7.9190,22.3000,0.0338,-0.2994,0.0184,-0.981388962,-0.616865309,267.067890648,0.4364,0.2961,0.5771,0.1123,0.0925,0.0784,0.0961,0.1009,5.1135,0f000001,0*21baf340\n\t", "INSPVAXA,USB3,0,50.0,FINESTEERING,2107,283639.700,02000000,471d,15824;INS_ALIGNMENT_COMPLETE,INS_RTKFIXED,37.37126158948,126.72209911436,7.9198,22.3000,0.0295,-0.3287,0.0146,-1.013704154,-0.682043166,267.265330343,0.4364,0.2961,0.5771,0.1123,0.0925,0.0784,0.0961,0.1009,5.1135,0f000001,0*ee73127b\n\t", "INSPVAXA,USB3,0,49.5,FINESTEERING,2107,283640.200,02000000,471d,15824;INS_ALIGNMENT_COMPLETE,INS_RTKFIXED,37.37126161750,126.72209746371,7.9213,22.3000,0.0430,-0.3344,0.0134,-0.961284284,-0.929903840,267.457563863,0.4362,0.2958,0.5770,0.1123,0.0925,0.0784,0.0961,0.1009,5.1150,0f000001,0*e2e7a72b\n\t", "INSPVAXA,USB3,0,49.5,FINESTEERING,2107,283640.700,02000000,471d,15824;INS_ALIGNMENT_COMPLETE,INS_RTKFIXED,37.37126164969,126.72209583664,7.9226,22.3000,0.0427,-0.3200,0.0053,-1.010366927,-1.135102181,267.635350069,0.4362,0.2958,0.5770,0.1123,0.0925,0.0784,0.0961,0.1009,5.1150,0f000001,0*6b674dca\n\t", "DUALANTENNAHEADINGA,USB3,0,50.0,FINESTEERING,2107,283641.200,02000000,d426,15824;INSUFFICIENT_OBS,NONE,-1.000000000,0.000000000,0.000000000,0.0,0.000000000,0.000000000,\"631T\",11,4,4,3,04,00,20,02*472a6cda\n\t", "INSPVAXA,USB3,0,50.0,FINESTEERING,2107,283641.700,02000000,471d,15824;INS_ALIGNMENT_COMPLETE,INS_RTKFIXED,37.37126176584,126.72209246619,7.9228,22.3000,0.0335,-0.3477,0.0031,-0.698463635,-1.495934209,267.964863954,0.4360,0.2957,0.5769,0.1125,0.0925,0.0784,0.0961,0.1009,5.1165,0f000001,0*ca9d9e5e\n\t", "INSPVAXA,USB3,0,50.0,FINESTEERING,2107,283642.200,02000000,471d,15824;INS_ALIGNMENT_COMPLETE,INS_RTKFIXED,37.37126183344,126.72209071714,7.9215,22.3000,0.0370,-0.3263,0.0036,-0.535216936,-1.667310153,268.031771555,0.4354,0.2957,0.5768,0.1127,0.0926,0.0784,0.0961,0.1009,5.1177,0f000001,0*11bec665\n\t", "DUALANTENNAHEADINGA,USB3,0,50.0,FINESTEERING,2107,283642.700,02000000,d426,15824;INSUFFICIENT_OBS,NONE,-1.000000000,0.000000000,0.000000000,0.0,0.000000000,0.000000000,\"631T\",12,4,4,3,04,00,20,03*f200c6d7\n\t", "DUALANTENNAHEADINGA,USB3,0,50.5,FINESTEERING,2107,283643.200,02000000,d426,15824;INSUFFICIENT_OBS,NONE,-1.000000000,0.000000000,0.000000000,0.0,0.000000000,0.000000000,\"631T\",14,4,4,3,04,00,20,02*f76a0e1e\n\t", "INSPVAXA,USB3,0,50.5,FINESTEERING,2107,283643.700,02000000,471d,15824;INS_ALIGNMENT_COMPLETE,INS_RTKFIXED,37.37126202513,126.72208597859,7.9183,22.3000,0.0299,-0.3163,0.0088,-0.418582783,-1.196326458,268.184941514,0.4349,0.2958,0.5767,0.1124,0.0926,0.0784,0.0961,0.1010,5.1181,0f000001,0*962e1d48\n\t", "INSPVAXA,USB3,0,50.0,FINESTEERING,2107,283644.200,02000000,471d,15824;INS_ALIGNMENT_COMPLETE,INS_RTKFIXED,37.37126209425,126.72208434200,7.9172,22.3000,0.0360,-0.2950,0.0056,-0.334802719,-0.884110622,268.233385323,0.4347,0.2959,0.5767,0.1122,0.0926,0.0784,0.0961,0.1010,5.1180,0f000001,0*78a9edf8\n\t", "INSPVAXA,USB3,0,50.0,FINESTEERING,2107,283644.700,02000000,471d,15824;INS_ALIGNMENT_COMPLETE,INS_RTKFIXED,37.37126215178,126.72208275426,7.9159,22.3000,0.0303,-0.2952,0.0021,-0.296302250,-0.633495852,268.293666475,0.4347,0.2959,0.5767,0.1122,0.0926,0.0784,0.0961,0.1010,5.1180,0f000001,0*8db6baa1\n\t", "INSPVAXA,USB3,0,46.0,FINESTEERING,2107,283645.200,02000000,471d,15824;INS_ALIGNMENT_COMPLETE,INS_RTKFIXED,37.37126220166,126.72208110110,7.9146,22.3000,0.0357,-0.3070,0.0007,-0.345507272,-0.608999756,268.311610368,0.4352,0.2960,0.5768,0.1123,0.0926,0.0784,0.0961,0.1011,5.1185,0f000001,0*f711e95a\n\t", "DUALANTENNAHEADINGA,USB3,0,46.0,FINESTEERING,2107,283645.700,02000000,d426,15824;INSUFFICIENT_OBS,NONE,-1.000000000,0.000000000,0.000000000,0.0,0.000000000,0.000000000,\"631T\",14,4,4,3,04,00,20,03*e6910734\n\t", "INSPVAXA,USB3,0,45.5,FINESTEERING,2107,283646.200,02000000,471d,15824;INS_ALIGNMENT_COMPLETE,INS_RTKFIXED,37.37126228996,126.72207792557,7.9145,22.3000,0.0424,-0.3064,0.0070,-0.583777876,-0.970443227,268.202528664,0.4357,0.2960,0.5768,0.1124,0.0925,0.0784,0.0961,0.1011,5.1194,0f000001,0*211ff137\n\t", "INSPVAXA,USB3,0,45.5,FINESTEERING,2107,283646.700,02000000,471d,15824;INS_ALIGNMENT_COMPLETE,INS_RTKFIXED,37.37126233833,126.72207631349,7.9144,22.3000,0.0451,-0.2992,0.0137,-0.600671632,-1.104685881,268.101292386,0.4357,0.2960,0.5768,0.1124,0.0925,0.0784,0.0961,0.1011,5.1194,0f000001,0*24418ec0\n\t", "DUALANTENNAHEADINGA,USB3,0,48.5,FINESTEERING,2107,283647.200,02000000,d426,15824;INSUFFICIENT_OBS,NONE,-1.000000000,0.000000000,0.000000000,0.0,0.000000000,0.000000000,\"631T\",13,4,4,3,04,00,20,03*e3593a63\n\t", "INSPVAXA,USB3,0,48.5,FINESTEERING,2107,283647.700,02000000,471d,15824;INS_ALIGNMENT_COMPLETE,INS_RTKFIXED,37.37126242655,126.72207309668,7.9156,22.3000,0.0394,-0.3060,0.0118,-0.639679760,-1.236455959,267.822984990,0.4363,0.2960,0.5769,0.1123,0.0925,0.0784,0.0961,0.1011,5.1206,0f000001,0*6bb51677\n\t", "INSPVAXA,USB3,0,48.0,FINESTEERING,2107,283648.200,02008000,471d,15824;INS_ALIGNMENT_COMPLETE,INS_RTKFIXED,37.37126246801,126.72207154325,7.9155,22.3000,0.0354,-0.2935,0.0108,-0.510675062,-1.137543161,267.571098751,0.4364,0.2959,0.5770,0.1124,0.0925,0.0784,0.0961,0.1011,5.1221,0f000001,0*c4dadb2f\n\t", "INSPVAXA,USB3,0,48.0,FINESTEERING,2107,283648.700,02008000,471d,15824;INS_ALIGNMENT_COMPLETE,INS_RTKFIXED,37.37126248707,126.72206994787,7.9152,22.3000,0.0198,-0.2907,0.0205,-0.532213630,-1.121566976,267.351964744,0.4364,0.2959,0.5770,0.1124,0.0925,0.0784,0.0961,0.1011,5.1221,0f000001,0*5feed5da\n\t", "INSPVAXA,USB3,0,50.5,FINESTEERING,2107,283649.200,02008000,471d,15824;INS_ALIGNMENT_COMPLETE,INS_RTKFIXED,37.37126248971,126.72206839810,7.9149,22.3000,0.0089,-0.2933,0.0096,-0.659725734,-0.970229399,267.160180872,0.4369,0.2958,0.5772,0.1125,0.0925,0.0784,0.0961,0.1011,5.1235,0f000001,0*081a7c85\n\t", "INSPVAXA,USB3,0,50.5,FINESTEERING,2107,283649.700,02008000,471d,15824;INS_ALIGNMENT_COMPLETE,INS_RTKFIXED,37.37126248182,126.72206686817,7.9130,22.3000,0.0195,-0.2818,0.0147,-0.676677557,-0.877493738,266.924781860,0.4369,0.2958,0.5772,0.1125,0.0925,0.0784,0.0961,0.1011,5.1235,0f000001,0*7b64dc48\n\t", "INSPVAXA,USB3,0,51.0,FINESTEERING,2107,283650.200,02008000,471d,15824;INS_ALIGNMENT_COMPLETE,INS_RTKFIXED,37.37126249199,126.72206547845,7.9115,22.3000,0.0164,-0.3260,0.0139,-0.484645802,-0.829453687,266.635151565,0.4374,0.2957,0.5772,0.1135,0.0925,0.0784,0.0961,0.1011,5.1243,0f000001,0*b0320f40\n\t", "INSPVAXA,USB3,0,51.0,FINESTEERING,2107,283650.700,02008000,471d,15824;INS_ALIGNMENT_COMPLETE,INS_RTKFIXED,37.37126248591,126.72206385137,7.9107,22.3000,0.0102,-0.2983,0.0161,-0.427862387,-0.984462668,266.224829667,0.4374,0.2957,0.5772,0.1135,0.0925,0.0784,0.0961,0.1011,5.1243,0f000001,0*ccab10f5\n\t", "INSPVAXA,USB3,0,46.5,FINESTEERING,2107,283651.200,02008000,471d,15824;INS_ALIGNMENT_COMPLETE,INS_RTKFIXED,37.37126247297,126.72206225341,7.9105,22.3000,-0.0025,-0.2931,0.0133,-0.399154165,-1.231884130,265.791711510,0.4388,0.2958,0.5773,0.1125,0.0926,0.0784,0.0961,0.1010,5.1233,0f000001,0*02f453ca\n\t", "DUALANTENNAHEADINGA,USB3,0,46.5,FINESTEERING,2107,283651.700,02008000,d426,15824;INSUFFICIENT_OBS,NONE,-1.000000000,0.000000000,0.000000000,0.0,0.000000000,0.000000000,\"631T\",12,4,4,3,04,00,20,02*dcd0f98d\n\t", "DUALANTENNAHEADINGA,USB3,0,52.0,FINESTEERING,2107,283652.200,02000000,d426,15824;INSUFFICIENT_OBS,NONE,-1.000000000,0.000000000,0.000000000,0.0,0.000000000,0.000000000,\"631T\",13,4,4,3,04,00,20,03*c51a48ea\n\t", "INSPVAXA,USB3,0,52.0,FINESTEERING,2107,283652.700,02000000,471d,15824;INS_ALIGNMENT_COMPLETE,INS_RTKFIXED,37.37126238850,126.72205745647,7.9080,22.3000,0.0144,-0.2874,0.0010,-0.261960509,-1.758395569,264.562436767,0.4386,0.2958,0.5773,0.1122,0.0925,0.0784,0.0961,0.1009,5.1223,0f000001,0*48b75177\n\t", "DUALANTENNAHEADINGA,USB3,0,49.5,FINESTEERING,2107,283653.200,02000000,d426,15824;INSUFFICIENT_OBS,NONE,-1.000000000,0.000000000,0.000000000,0.0,0.000000000,0.000000000,\"631T\",12,4,4,3,04,00,20,02*b48bfb58\n\t", "DUALANTENNAHEADINGA,USB3,0,49.5,FINESTEERING,2107,283653.700,02000000,d426,15824;INSUFFICIENT_OBS,NONE,-1.000000000,0.000000000,0.000000000,0.0,0.000000000,0.000000000,\"631T\",11,4,4,3,04,00,20,03*b7c95c3e\n\t", "DUALANTENNAHEADINGA,USB3,0,45.0,FINESTEERING,2107,283654.200,02000000,d426,15824;INSUFFICIENT_OBS,NONE,-1.000000000,0.000000000,0.000000000,0.0,0.000000000,0.000000000,\"631T\",11,4,4,3,04,00,20,03*317f5696\n\t", "DUALANTENNAHEADINGA,USB3,0,45.0,FINESTEERING,2107,283654.700,02000000,d426,15824;INSUFFICIENT_OBS,NONE,-1.000000000,0.000000000,0.000000000,0.0,0.000000000,0.000000000,\"631T\",12,4,4,3,04,00,20,03*453ac166\n\t", "DUALANTENNAHEADINGA,USB3,0,47.5,FINESTEERING,2107,283655.200,02000000,d426,15824;INSUFFICIENT_OBS,NONE,-1.000000000,0.000000000,0.000000000,0.0,0.000000000,0.000000000,\"631T\",13,4,4,3,04,00,20,02*c2e72fac\n\t", "DUALANTENNAHEADINGA,USB3,0,47.5,FINESTEERING,2107,283655.700,02000000,d426,15824;INSUFFICIENT_OBS,NONE,-1.000000000,0.000000000,0.000000000,0.0,0.000000000,0.000000000,\"631T\",11,4,4,3,04,00,20,03*16470892\n\t", "DUALANTENNAHEADINGA,USB3,0,50.0,FINESTEERING,2107,283656.200,02000000,d426,15824;INSUFFICIENT_OBS,NONE,-1.000000000,0.000000000,0.000000000,0.0,0.000000000,0.000000000,\"631T\",11,4,4,3,04,00,20,02*6231c6e0\n\t",
